vi "Convert_to_time_between_Samples.vi"(1 "LDA 1st Group in":dbl[][](array[numeric])) -> (0 "LDA 1st Group out":dbl[][](array[numeric]))   [LabVIEW 2013]
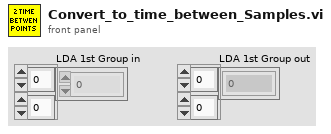
[diagram p1: front panel]
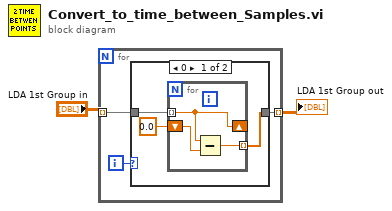
[diagram p0: block diagram]
diagram:
  n1 = for {
    tunnel: "LDA 1st Group in" -> [w4] mode=indexing
    tunnel: [w3] -> w2 mode=indexing
    i -> [w5]
    n2 = case shown="0" w5 {
      tunnel: w4 -> [w8 w12]
      tunnel: [w6 w12] -> w3
      frame 0 {
        n3 = for {
          shift-right: [w10] -> _
          shift-left: 0.0 ("Numeric") -> [w11]
          tunnel: w8 -> [w10] mode=indexing
          tunnel: [w9] -> w6 mode=indexing
          n4 = Subtract(x=w10, y=w11) -> (x-y=w9:dbl)
        }
      }
      frame 1, Default {
      }
    }
  }
  "LDA 1st Group out" <- w2
